vi "Next_Core.vi"(8 "error in (no error)":errorcluster, 10 "Query in":refnum<class "ADOResult.lvclass">, 11 "SqlMapper in":refnum<class "SqlMapper.lvclass">) -> (0 "error out":errorcluster, 1 "found?":bool=TRUE, 2 "Row":variant, 3 "SqlMapper out":refnum<class "SqlMapper.lvclass">)   [LabVIEW 2020, in "ORM_ADONet.lvlib" / "ADOResult.lvclass"]
uses:
  ADOResult.lvclass
  <vilib>/Viviota/shared/ORM.lvlibp/ORM/SqlMapper/SqlMapper.lvclass
  ADOResult.lvclass/ADOResult.ctl
  Read Reader.vi
  System.Data
  ADORow/ADORow.lvclass
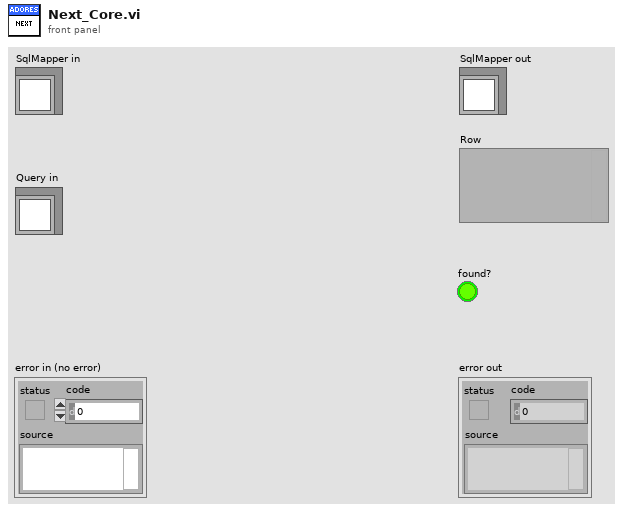
[diagram p1: front panel]
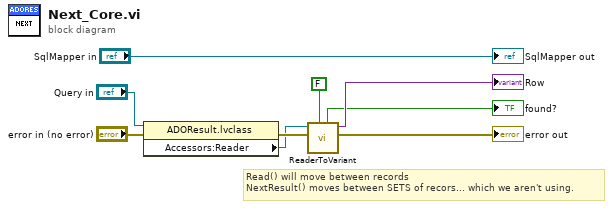
[diagram p0: block diagram]
diagram:
  # "Read() will move between records\nNextResult() moves between SETS of recors... which we aren't using."
  n1 = property class="ADOResult.lvclass"(reference="Query in", error in="error in (no error)") -> (error out=w3:errorcluster, "Accessors:Reader"=w1:refnum<k24>)  [unwired: 1 out]
  n2 = call "ReaderToVariant.vi"("CloseReader"=FALSE, "Error In"=w3, "Reader"=w1) -> ("Error Out"=→"error out":errorcluster, "Variant"=→"Row":variant, "Read"=→"found?":bool)  [unwired: 6 in]
  "SqlMapper out" <- "SqlMapper in"
